vi "Open-Close.vi"(5 "Username":string, 6 "Password":string, 7 "Address":string, 8 "Error In":errorcluster) -> (0 "Error Out":errorcluster)   [LabVIEW 2018, in "Tests.lvlib" / "SFTP File.lvlib"]
uses:
  SFTP File.lvlib
  src/Toolkit/SFTP File/Type Definitions/Open Options.ctl
  src/Toolkit/SFTP File/Support/Open from SFTP.vi
  src/Toolkit/SFTP File/Support/Close to SFTP.vi
  <vilib>/addons/_JKI Toolkits/Caraya/classes/Test/Test.lvclass
  <vilib>/addons/_JKI Toolkits/Caraya/classes/Assert/Assert.lvclass
  src/Toolkit/SFTP File/SFTP File.lvclass
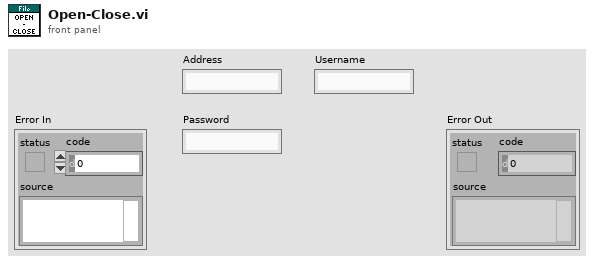
[diagram p1: front panel]
types:
  T1 = typedef "Toolkit.lvlib/SFTP File.lvclass/Open Options.ctl" = cluster{"Read":bool, "Write":bool, "Append":bool, "Create":bool, "Truncate":bool, "Exclude":bool}
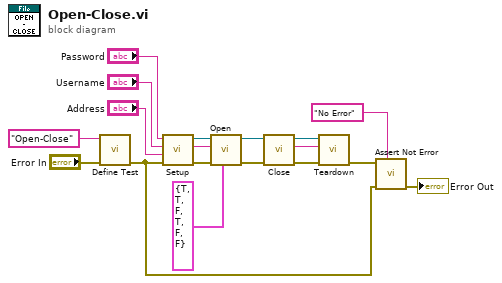
[diagram p0: block diagram]
diagram:
  n1 = call <vilib>:"Define Test.vi"("error in (no error)"="Error In", "Label (VI Title)"="Open-Close") -> ("error out"=w14:errorcluster)  [unwired: 9 in]
  n2 = call "Setup.vi"("Error In"=w14, "Password"="Address", "Username"="Username", "Address"="Password") -> ("Error Out"=w5:errorcluster, "Temporary File"=w4:string, "SFTP"=w7:refnum<class "SFTP.lvclass">)  [unwired: 5 in]
  n3 = call-poly "Open.vi"("Options"=T1 {"Read"=TRUE, "Write"=TRUE, "Append"=FALSE, "Create"=TRUE, "Truncate"=FALSE, "Exclude"=FALSE} ("Flags"), "Error In"=w5, "Remote Path"=w4, "SFTP"=w7) -> ("Error Out"=w10:errorcluster, "SFTP File"=w11:refnum<class "SFTP File.lvclass">)  [unwired: 6 in]
  n4 = call-poly "Close.vi"("Error In"=w10, "SFTP File"=w11) -> ("Error Out"=w1:errorcluster, "Remote Path"=w2:string, "SFTP"=w3:refnum<class "SFTP.lvclass">)  [unwired: 7 in]
  n5 = call "Teardown.vi"("Error In"=w1, "Temporary File"=w2, "SFTP"=w3) -> ("Error Out"=w16:errorcluster)  [unwired: 8 in]
  n6 = call <vilib>:"Assert Not Error.vi"("Label"="No Error", "error in (no error)"=w14, "Not Error?"=w16) -> ("error out"=→"Error Out":errorcluster)  [unwired: 8 in]
